vi "Spy Check Last Specific Message Received.vi"(8 "error in (no error)":errorcluster, 10 "Specific Call":string, 11 "Mock Rig Process In":refnum<class "Mock Process.lvclass">) -> (0 "error out":errorcluster, 1 "Message Data":variant, 2 "Messages":string[](array[string]), 3 "Mock Rig Process Out":refnum<class "Mock Process.lvclass">)   [LabVIEW 2020, in "Mock Process.lvclass"]
uses:
  Mock Process.lvclass
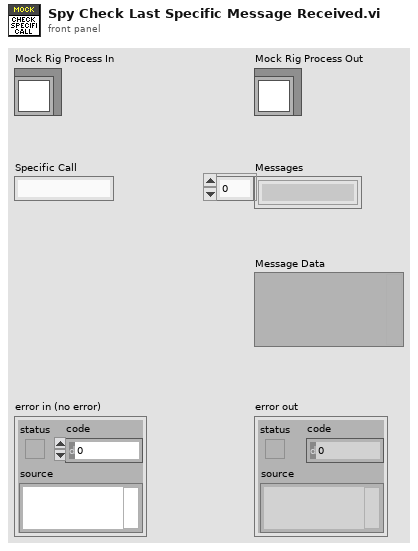
[diagram p1: front panel]
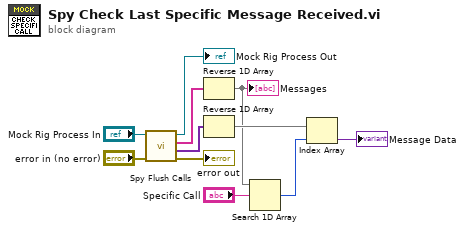
[diagram p0: block diagram]
diagram:
  n1 = call "Spy Flush Calls.vi"("error in (no error)"="error in (no error)", "Mock Process In"="Mock Rig Process In") -> ("error out"=→"error out":errorcluster, "Message Data"=w1:variant[], "Message"=w2:string[], "Mock Process Out"=→"Mock Rig Process Out":refnum<class "Mock Process.lvclass">)  [unwired: 6 in]
  n2 = Reverse 1D Array(array=w2) -> (reversed array=w4:string[])
  "Messages" <- w4
  n3 = Reverse 1D Array(array=w1) -> (reversed array=w5:variant[])
  n4 = Search 1D Array(1D array=w4, element="Specific Call") -> (index of element=w7:i32)  [unwired: 1 in]
  n5 = Index Array(array=w5, index=w7) -> (element=→"Message Data":variant)
